vi "Remove Duplicate Enqueuer.vi"(11 "Enqueuers in":refnum<class "Message Enqueuer.lvclass">[](array[class])) -> (3 "Unique Enqueuers out":refnum<class "Message Enqueuer.lvclass">[](array[class]))   [LabVIEW 2020]
doc: "Remove all duplicate enqueuers from 'Enqueuers in'.\n\nDeprecated: Replace with content."
uses:
  PPL/HDH.Actor Framework.Core.Actor.lvlibp/1abvi3w/vi.lib/ActorFramework/Message Enqueuer/Message Enqueuer.lvclass
  4e7ddeb3-a944-47ef-8a2f-21134f5781d7.vi
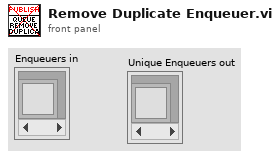
[diagram p1: front panel]
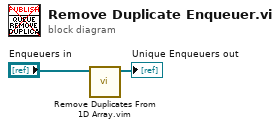
[diagram p0: block diagram]
diagram:
  n1 = call "Remove Duplicates From 1D Array.vim"("array"="Enqueuers in") -> ("array with duplicates removed"=→"Unique Enqueuers out":refnum<class "Message Enqueuer.lvclass">[])  [unwired: 10 in]
